vi "Autonomous Independent.vi"() -> ()   [LabVIEW 2015]
doc: "This VI is called when autonomous begins, and will automatically be terminated when autonomous ends. You can carry out timed or sensor driven robot movement independently without needing to return to the caller."
uses:
  Robot Global Data.vi
  <vilib>/Rock Robotics/Network Tables/NT Read Number.vi
panel:
  out "Stuck?":bool
  out "Position":dbl
  out "Temporary Center":dbl
  # "Be sure to right-click and choose Data Operations>>Make Current Value default if you want to save the array values with the VI"
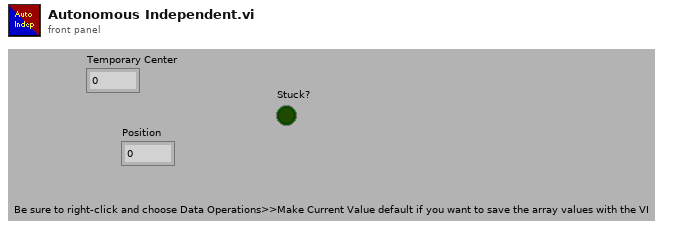
[diagram p1: front panel]
types:
  T1 = cluster{"Numeric":dbl, "Numeric":dbl, dbl, dbl, "Numeric":dbl, "Numeric":dbl}[]
  T2 = cluster{"Numeric":dbl, "Numeric":dbl, dbl, dbl, "Numeric":dbl, "Numeric":dbl}
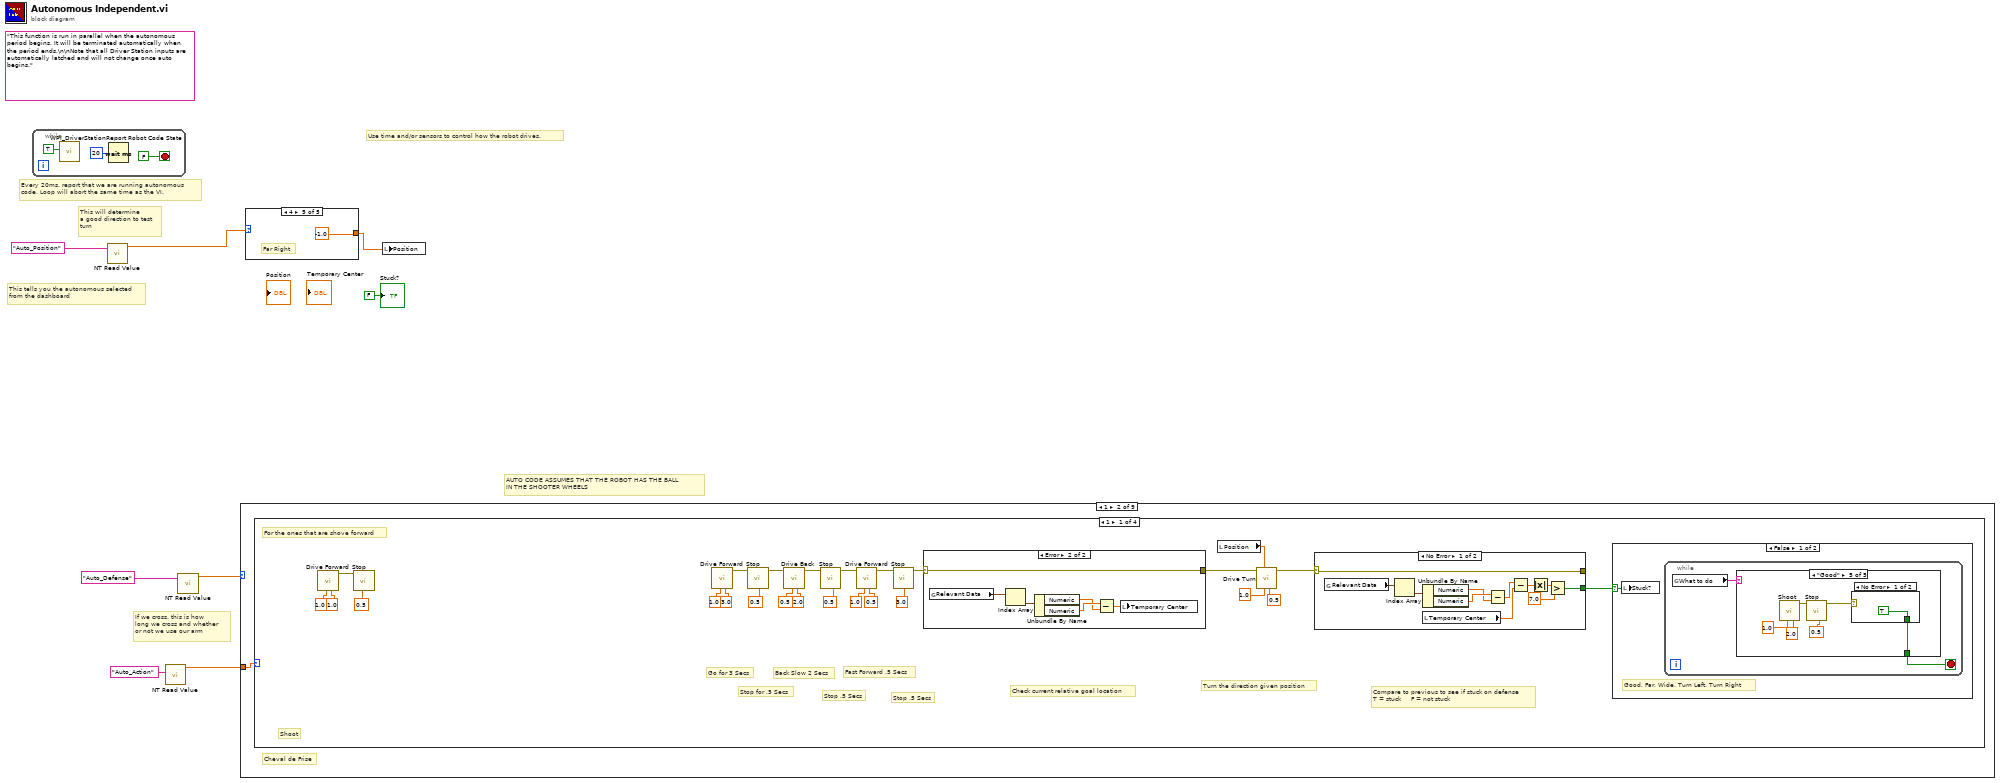
[diagram p0: block diagram]
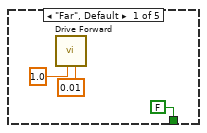
[diagram p3: hidden frame]
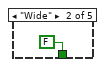
[diagram p4: hidden frame]
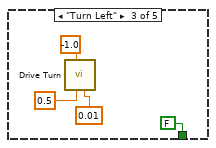
[diagram p5: hidden frame]
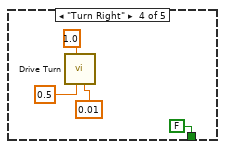
[diagram p6: hidden frame]
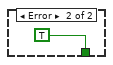
[diagram p7: hidden frame]
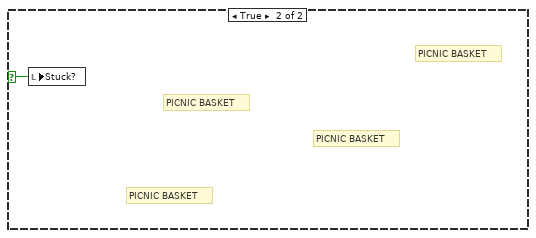
[diagram p8: hidden frame]
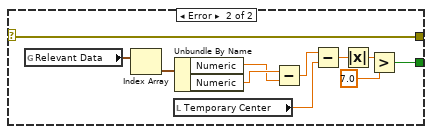
[diagram p9: hidden frame]
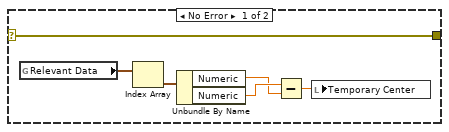
[diagram p10: hidden frame]
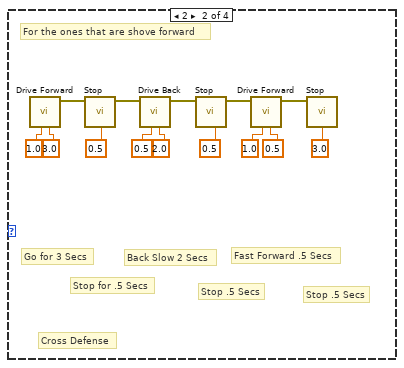
[diagram p11: hidden frame]
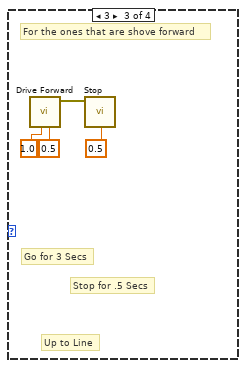
[diagram p12: hidden frame]
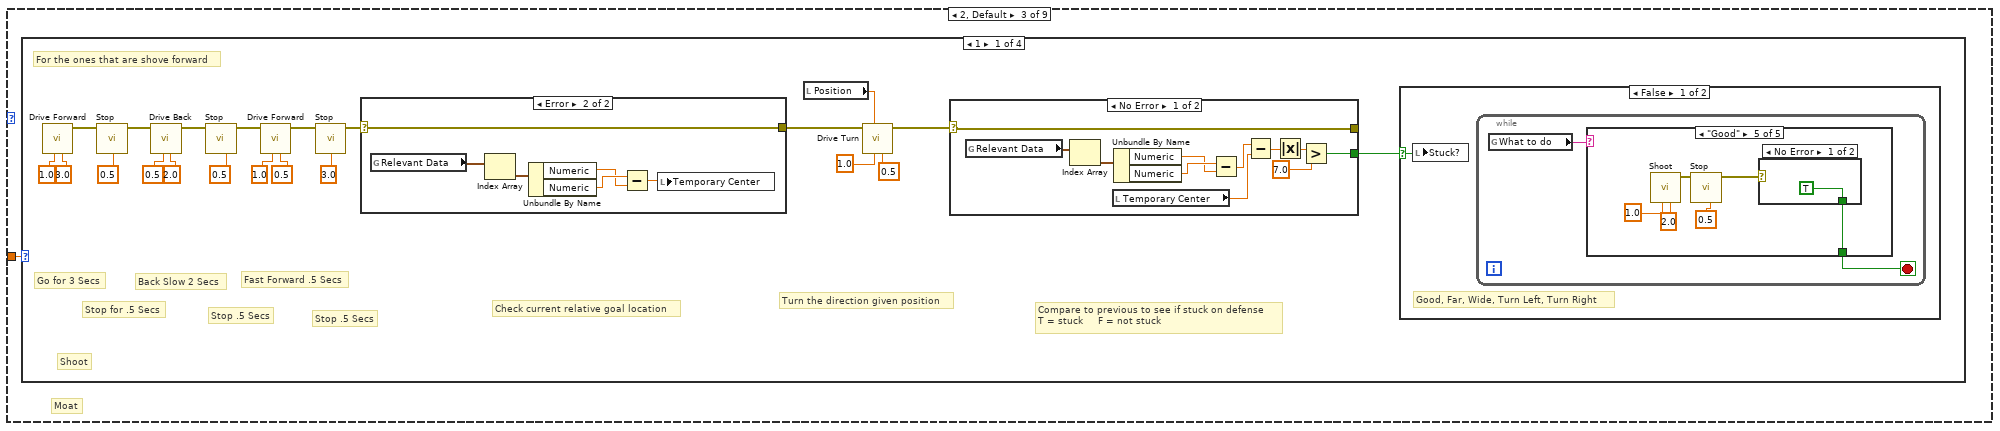
[diagram p14: hidden frame]
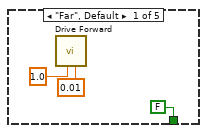
[diagram p15: hidden frame]
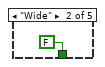
[diagram p16: hidden frame]
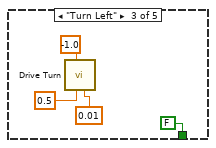
[diagram p17: hidden frame]
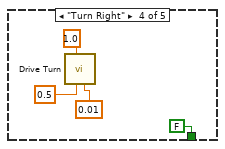
[diagram p18: hidden frame]
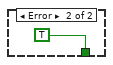
[diagram p19: hidden frame]
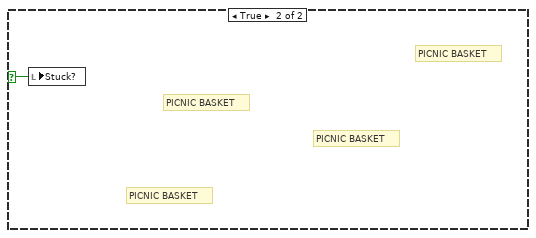
[diagram p20: hidden frame]
diagram:
  (unwired) "This function is run in parallel when the autonomous period begins. It will be terminated automatically when the period ends.\n\nNote that all Driver Station inputs are automatically latched and will not change once auto begins."
  # "AUTO CODE ASSUMES THAT THE ROBOT HAS THE BALL\nIN THE SHOOTER WHEELS"
  # "If we cross, this is how\nlong we cross and whether \nor not we use our arm"
  # "This will determine\na good direction to test\nturn"
  # "This tells you the autonomous selected\nfrom the dashboard"
  # "Every 20ms, report that we are running autonomous\ncode. Loop will abort the same time as the VI."
  # "Use time and/or sensors to control how the robot drives."
  n1 = while {
    stop <- FALSE stop-if-true
    n2 = call <vilib>:"WPI_DriverStationReport Robot Code State.vi"("Autonomous"=TRUE) -> ()  [unwired: 10 in, 1 out]
    n3 = Wait (ms)(milliseconds to wait=u32 20) -> ()  [unwired: 1 out]
  }
  n4 = call-poly <vilib>:"NT Read Value.vi"("Name"="Auto_Position") -> ("Numeric"=w7:dbl)  [unwired: 9 in, 1 out]
  n5 = call-poly <vilib>:"NT Read Value.vi"("Name"="Auto_Action") -> ("Numeric"=w1:dbl)  [unwired: 9 in, 1 out]
  n6 = call-poly <vilib>:"NT Read Value.vi"("Name"="Auto_Defense") -> ("Numeric"=w6:dbl)  [unwired: 9 in, 1 out]
  n7 = case shown="1" w6 {
    tunnel: w1 -> [_ w12 w114 _ _ _ _ _ _]
    frame 0 {
      # "Portcullis"
    }
    frame 1 {
      # "Cheval de Frise"
      n8 = case shown="1" w12 {
        frame 1 {
          # "Shoot"
          # "Check current relative goal location"
          # "Stop .5 Secs"
          # "Turn the direction given position"
          # "Compare to previous to see if stuck on defense\nT = stuck     F = not stuck"
          # "Fast Forward .5 Secs"
          # "Stop .5 Secs"
          # "Back Slow 2 Secs"
          # "Stop for .5 Secs"
          # "Go for 3 Secs"
          # "For the ones that are shove forward"
          n9 = call "Drive Forward.vi"("Time"=1.0, "Speed"=1.0) -> ("error out"=w13:errorcluster)  [unwired: 9 in]
          n10 = call "Stop.vi"("Time"=0.5, "error in"=w13) -> ()  [unwired: 9 in, 1 out]
          n11 = call "Drive Forward.vi"("Time"=3.0, "Speed"=1.0) -> ("error out"=w37:errorcluster)  [unwired: 9 in]
          n12 = call "Stop.vi"("Time"=0.5, "error in"=w37) -> ("error out"=w36:errorcluster)  [unwired: 9 in]
          n13 = call "Drive Back.vi"("Time"=2.0, "Speed"=0.5, "error in"=w36) -> ("error out"=w35:errorcluster)  [unwired: 8 in]
          n14 = call "Stop.vi"("Time"=0.5, "error in"=w35) -> ("error out"=w34:errorcluster)  [unwired: 9 in]
          n15 = call "Drive Forward.vi"("Time"=0.5, "Speed"=1.0, "error in"=w34) -> ("error out"=w33:errorcluster)  [unwired: 8 in]
          n16 = call "Stop.vi"("Time"=3.0, "error in"=w33) -> ("error out"=w23:errorcluster)  [unwired: 9 in]
          n17 = case shown="Error" w23 {
            selector: w23 -> [w84 w90]
            tunnel: [w84 w90] -> w22
            frame No Error {
              n18 = global read "Robot Global Data.vi" "Relevant Data"() -> (w89:T1)
              n19 = Index Array(array=w89) -> (element=w88:T2)  [unwired: 1 in]
              n20 = Unbundle By Name(w88) -> ("Numeric"=w86:dbl, "Numeric"=w87:dbl)
              n21 = Subtract(x=w87, y=w86) -> (x-y=w85:dbl)
              n22 = local write "Temporary Center"(w85) -> ()
            }
            frame Error {
              n23 = global read "Robot Global Data.vi" "Relevant Data"() -> (w95:T1)
              n24 = Index Array(array=w95) -> (element=w94:T2)  [unwired: 1 in]
              n25 = Unbundle By Name(w94) -> ("Numeric"=w92:dbl, "Numeric"=w93:dbl)
              n26 = Subtract(x=w93, y=w92) -> (x-y=w91:dbl)
              n27 = local write "Temporary Center"(w91) -> ()
            }
          }
          n28 = local read "Position"() -> (w21:dbl)
          n29 = call "Drive Turn.vi"("Time"=0.5, "Speed"=1.0, "Direction"=w21, "error in"=w22) -> ("error out"=w18:errorcluster)  [unwired: 7 in]
          n30 = case shown="No Error" w18 {
            selector: w18 -> [w68 w79]
            tunnel: [w68 w79] -> _
            tunnel: [w62 w73] -> w17
            frame No Error {
              n31 = global read "Robot Global Data.vi" "Relevant Data"() -> (w72:T1)
              n32 = Index Array(array=w72) -> (element=w71:T2)  [unwired: 1 in]
              n33 = local read "Temporary Center"() -> (w66:dbl)
              n34 = Unbundle By Name(w71) -> ("Numeric"=w69:dbl, "Numeric"=w70:dbl)
              n35 = Subtract(x=w70, y=w69) -> (x-y=w67:dbl)
              n36 = Subtract(x=w67, y=w66) -> (x-y=w65:dbl)
              n37 = Absolute Value(x=w65) -> (abs(x)=w64:dbl)
              n38 = Greater?(x=w64, y=7.0) -> (0:w62:bool)
            }
            frame Error {
              n39 = global read "Robot Global Data.vi" "Relevant Data"() -> (w83:T1)
              n40 = Index Array(array=w83) -> (element=w82:T2)  [unwired: 1 in]
              n41 = local read "Temporary Center"() -> (w77:dbl)
              n42 = Unbundle By Name(w82) -> ("Numeric"=w80:dbl, "Numeric"=w81:dbl)
              n43 = Subtract(x=w81, y=w80) -> (x-y=w78:dbl)
              n44 = Subtract(x=w78, y=w77) -> (x-y=w76:dbl)
              n45 = Absolute Value(x=w76) -> (abs(x)=w75:dbl)
              n46 = Greater?(x=w75, y=7.0) -> (0:w73:bool)
            }
          }
          n47 = case shown="False" w17 {
            selector: w17 -> [w38 w61]
            frame False {
              # "Good, Far, Wide, Turn Left, Turn Right"
              n48 = local write "Stuck?"(w38) -> ()
              n49 = while {
                stop <- w39 stop-if-true
                n50 = global read "Robot Global Data.vi" "What to do"() -> (w40:string)
                n51 = case shown="\"Good\"" w40 {
                  tunnel: [FALSE FALSE FALSE FALSE w53] -> w39
                  frame "Far", Default {
                    n52 = call "Drive Forward.vi"("Time"=0.01, "Speed"=1.0) -> ()  [unwired: 9 in, 1 out]
                  }
                  frame "Wide" {
                  }
                  frame "Turn Left" {
                    n53 = call "Drive Turn.vi"("Time"=0.01, "Speed"=0.5, "Direction"=-1.0) -> ()  [unwired: 8 in, 1 out]
                  }
                  frame "Turn Right" {
                    n54 = call "Drive Turn.vi"("Time"=0.01, "Speed"=0.5, "Direction"=1.0) -> ()  [unwired: 8 in, 1 out]
                  }
                  frame "Good" {
                    n55 = call "Shoot.vi"("Time"=2.0, "Speed"=1.0) -> ("error out"=w56:errorcluster)  [unwired: 9 in]
                    n56 = call "Stop.vi"("Time"=0.5, "error in"=w56) -> ("error out"=w54:errorcluster)  [unwired: 9 in]
                    n57 = case shown="No Error" w54 {
                      tunnel: [TRUE TRUE] -> w53
                      frame No Error {
                      }
                      frame Error {
                      }
                    }
                  }
                }
              }
            }
            frame True {
              # "PICNIC BASKET"
              # "PICNIC BASKET"
              # "PICNIC BASKET"
              # "PICNIC BASKET"
              n58 = local write "Stuck?"(w61) -> ()
            }
          }
        }
        frame 2 {
          # "Cross Defense"
          # "Stop .5 Secs"
          # "Fast Forward .5 Secs"
          # "Stop .5 Secs"
          # "Back Slow 2 Secs"
          # "Stop for .5 Secs"
          # "Go for 3 Secs"
          # "For the ones that are shove forward"
          n59 = call "Drive Forward.vi"("Time"=3.0, "Speed"=1.0) -> ("error out"=w109:errorcluster)  [unwired: 9 in]
          n60 = call "Stop.vi"("Time"=0.5, "error in"=w109) -> ("error out"=w108:errorcluster)  [unwired: 9 in]
          n61 = call "Drive Back.vi"("Time"=2.0, "Speed"=0.5, "error in"=w108) -> ("error out"=w107:errorcluster)  [unwired: 8 in]
          n62 = call "Stop.vi"("Time"=0.5, "error in"=w107) -> ("error out"=w106:errorcluster)  [unwired: 9 in]
          n63 = call "Drive Forward.vi"("Time"=0.5, "Speed"=1.0, "error in"=w106) -> ("error out"=w105:errorcluster)  [unwired: 8 in]
          n64 = call "Stop.vi"("Time"=3.0, "error in"=w105) -> ()  [unwired: 9 in, 1 out]
        }
        frame 3 {
          # "Up to Line"
          # "Stop for .5 Secs"
          # "Go for 3 Secs"
          # "For the ones that are shove forward"
          n65 = call "Drive Forward.vi"("Time"=0.5, "Speed"=1.0) -> ("error out"=w113:errorcluster)  [unwired: 9 in]
          n66 = call "Stop.vi"("Time"=0.5, "error in"=w113) -> ()  [unwired: 9 in, 1 out]
        }
        frame 0, Default {
          # "Disabled"
        }
      }
    }
    frame 2, Default {
      # "Moat"
      n67 = case shown="1" w114 {
        frame 1 {
          # "Shoot"
          # "Check current relative goal location"
          # "Stop .5 Secs"
          # "Turn the direction given position"
          # "Compare to previous to see if stuck on defense\nT = stuck     F = not stuck"
          # "Fast Forward .5 Secs"
          # "Stop .5 Secs"
          # "Back Slow 2 Secs"
          # "Stop for .5 Secs"
          # "Go for 3 Secs"
          # "For the ones that are shove forward"
          n68 = call "Drive Forward.vi"("Time"=3.0, "Speed"=1.0) -> ("error out"=w135:errorcluster)  [unwired: 9 in]
          n69 = call "Stop.vi"("Time"=0.5, "error in"=w135) -> ("error out"=w134:errorcluster)  [unwired: 9 in]
          n70 = call "Drive Back.vi"("Time"=2.0, "Speed"=0.5, "error in"=w134) -> ("error out"=w133:errorcluster)  [unwired: 8 in]
          n71 = call "Stop.vi"("Time"=0.5, "error in"=w133) -> ("error out"=w132:errorcluster)  [unwired: 9 in]
          n72 = call "Drive Forward.vi"("Time"=0.5, "Speed"=1.0, "error in"=w132) -> ("error out"=w131:errorcluster)  [unwired: 8 in]
          n73 = call "Stop.vi"("Time"=3.0, "error in"=w131) -> ("error out"=w121:errorcluster)  [unwired: 9 in]
          n74 = case shown="Error" w121 {
            selector: w121 -> [w182 w188]
            tunnel: [w182 w188] -> w120
            frame No Error {
              n75 = global read "Robot Global Data.vi" "Relevant Data"() -> (w187:T1)
              n76 = Index Array(array=w187) -> (element=w186:T2)  [unwired: 1 in]
              n77 = Unbundle By Name(w186) -> ("Numeric"=w184:dbl, "Numeric"=w185:dbl)
              n78 = Subtract(x=w185, y=w184) -> (x-y=w183:dbl)
              n79 = local write "Temporary Center"(w183) -> ()
            }
            frame Error {
              n80 = global read "Robot Global Data.vi" "Relevant Data"() -> (w193:T1)
              n81 = Index Array(array=w193) -> (element=w192:T2)  [unwired: 1 in]
              n82 = Unbundle By Name(w192) -> ("Numeric"=w190:dbl, "Numeric"=w191:dbl)
              n83 = Subtract(x=w191, y=w190) -> (x-y=w189:dbl)
              n84 = local write "Temporary Center"(w189) -> ()
            }
          }
          n85 = local read "Position"() -> (w119:dbl)
          n86 = call "Drive Turn.vi"("Time"=0.5, "Speed"=1.0, "Direction"=w119, "error in"=w120) -> ("error out"=w116:errorcluster)  [unwired: 7 in]
          n87 = case shown="No Error" w116 {
            selector: w116 -> [w166 w177]
            tunnel: [w166 w177] -> _
            tunnel: [w160 w171] -> w115
            frame No Error {
              n88 = global read "Robot Global Data.vi" "Relevant Data"() -> (w170:T1)
              n89 = Index Array(array=w170) -> (element=w169:T2)  [unwired: 1 in]
              n90 = local read "Temporary Center"() -> (w164:dbl)
              n91 = Unbundle By Name(w169) -> ("Numeric"=w167:dbl, "Numeric"=w168:dbl)
              n92 = Subtract(x=w168, y=w167) -> (x-y=w165:dbl)
              n93 = Subtract(x=w165, y=w164) -> (x-y=w163:dbl)
              n94 = Absolute Value(x=w163) -> (abs(x)=w162:dbl)
              n95 = Greater?(x=w162, y=7.0) -> (0:w160:bool)
            }
            frame Error {
              n96 = global read "Robot Global Data.vi" "Relevant Data"() -> (w181:T1)
              n97 = Index Array(array=w181) -> (element=w180:T2)  [unwired: 1 in]
              n98 = local read "Temporary Center"() -> (w175:dbl)
              n99 = Unbundle By Name(w180) -> ("Numeric"=w178:dbl, "Numeric"=w179:dbl)
              n100 = Subtract(x=w179, y=w178) -> (x-y=w176:dbl)
              n101 = Subtract(x=w176, y=w175) -> (x-y=w174:dbl)
              n102 = Absolute Value(x=w174) -> (abs(x)=w173:dbl)
              n103 = Greater?(x=w173, y=7.0) -> (0:w171:bool)
            }
          }
          n104 = case shown="False" w115 {
            selector: w115 -> [w136 w159]
            frame False {
              # "Good, Far, Wide, Turn Left, Turn Right"
              n105 = local write "Stuck?"(w136) -> ()
              n106 = while {
                stop <- w137 stop-if-true
                n107 = global read "Robot Global Data.vi" "What to do"() -> (w138:string)
                n108 = case shown="\"Good\"" w138 {
                  tunnel: [FALSE FALSE FALSE FALSE w151] -> w137
                  frame "Far", Default {
                    n109 = call "Drive Forward.vi"("Time"=0.01, "Speed"=1.0) -> ()  [unwired: 9 in, 1 out]
                  }
                  frame "Wide" {
                  }
                  frame "Turn Left" {
                    n110 = call "Drive Turn.vi"("Time"=0.01, "Speed"=0.5, "Direction"=-1.0) -> ()  [unwired: 8 in, 1 out]
                  }
                  frame "Turn Right" {
                    n111 = call "Drive Turn.vi"("Time"=0.01, "Speed"=0.5, "Direction"=1.0) -> ()  [unwired: 8 in, 1 out]
                  }
                  frame "Good" {
                    n112 = call "Shoot.vi"("Time"=2.0, "Speed"=1.0) -> ("error out"=w154:errorcluster)  [unwired: 9 in]
                    n113 = call "Stop.vi"("Time"=0.5, "error in"=w154) -> ("error out"=w152:errorcluster)  [unwired: 9 in]
                    n114 = case shown="No Error" w152 {
                      tunnel: [TRUE TRUE] -> w151
                      frame No Error {
                      }
                      frame Error {
                      }
                    }
                  }
                }
              }
            }
            frame True {
              # "PICNIC BASKET"
              # "PICNIC BASKET"
              # "PICNIC BASKET"
              # "PICNIC BASKET"
              n115 = local write "Stuck?"(w159) -> ()
            }
          }
        }
        frame 2 {
          # "Cross Defense"
          # "Stop .5 Secs"
          # "Fast Forward .5 Secs"
          # "Stop .5 Secs"
          # "Back Slow 2 Secs"
          # "Stop for .5 Secs"
          # "Go for 3 Secs"
          # "For the ones that are shove forward"
          n116 = call "Drive Forward.vi"("Time"=3.0, "Speed"=1.0) -> ("error out"=w207:errorcluster)  [unwired: 9 in]
          n117 = call "Stop.vi"("Time"=0.5, "error in"=w207) -> ("error out"=w206:errorcluster)  [unwired: 9 in]
          n118 = call "Drive Back.vi"("Time"=2.0, "Speed"=0.5, "error in"=w206) -> ("error out"=w205:errorcluster)  [unwired: 8 in]
          n119 = call "Stop.vi"("Time"=0.5, "error in"=w205) -> ("error out"=w204:errorcluster)  [unwired: 9 in]
          n120 = call "Drive Forward.vi"("Time"=0.5, "Speed"=1.0, "error in"=w204) -> ("error out"=w203:errorcluster)  [unwired: 8 in]
          n121 = call "Stop.vi"("Time"=3.0, "error in"=w203) -> ()  [unwired: 9 in, 1 out]
        }
        frame 3 {
          # "Up to Line"
          # "Stop for .5 Secs"
          # "Go for 3 Secs"
          # "For the ones that are shove forward"
          n122 = call "Drive Forward.vi"("Time"=0.5, "Speed"=1.0) -> ("error out"=w211:errorcluster)  [unwired: 9 in]
          n123 = call "Stop.vi"("Time"=0.5, "error in"=w211) -> ()  [unwired: 9 in, 1 out]
        }
        frame 0, Default {
          # "Disabled"
        }
      }
    }
    frame 3 {
      # "Ramparts"
    }
    frame 4 {
      # "Drawbridge"
    }
    frame 5 {
      # "Sally Port"
    }
    frame 6 {
      # "Rock Wall"
    }
    frame 7 {
      # "Rough Terrain"
    }
    frame 8 {
      # "Low Bar"
    }
  }
  n124 = case shown="4" w7 {
    tunnel: [1.0 1.0 1.0 1.0 -1.0] -> w4
    frame 0 {
      # "Far Left"
    }
    frame 1 {
      # "Left"
    }
    frame 2, Default {
      # "Middle"
    }
    frame 3 {
      # "Right"
    }
    frame 4 {
      # "Far Right"
    }
  }
  n125 = local write "Position"(w4) -> ()
  "Stuck?" <- FALSE ("Stuck?")
